vi "Archery_Main.vi"() -> ()   [LabVIEW 2014]
panel:
  in  "Exit":bool
  in  "Cluster":T1
  # "Archery Simulator"
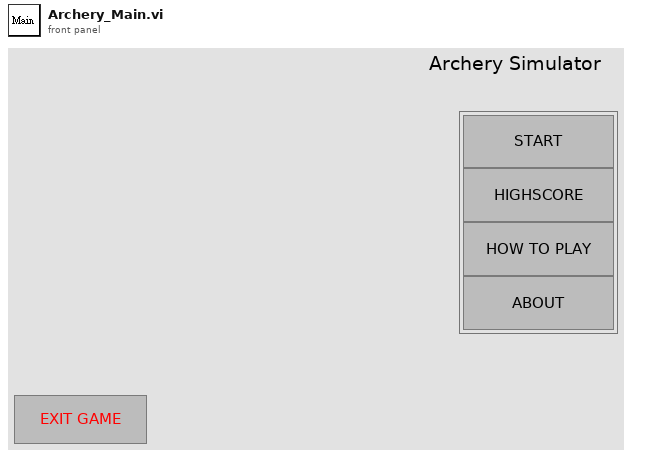
[diagram p1: front panel]
types:
  T1 = cluster{"Start":bool, "Highscore":bool, "Highscore 2":bool, "Highscore 3":bool}
  T2 = enum16{"init", "wait", "game", "highscore", "about", "hint"}
  T3 = enum16{"init", "wait", "game", "highscore", "about"}
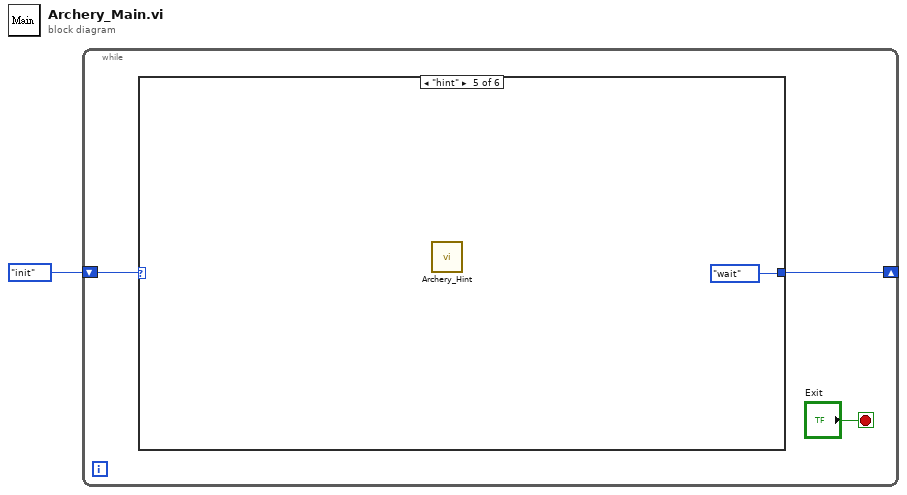
[diagram p0: block diagram]
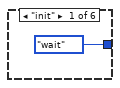
[diagram p2: hidden frame]
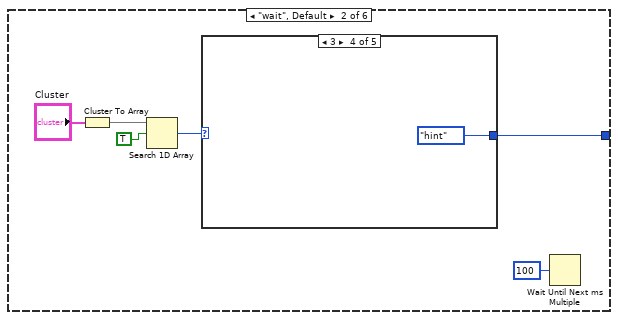
[diagram p3: hidden frame]
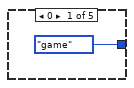
[diagram p4: hidden frame]
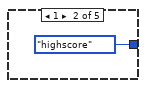
[diagram p5: hidden frame]
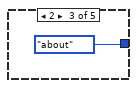
[diagram p6: hidden frame]
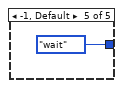
[diagram p7: hidden frame]
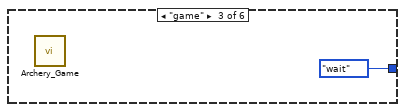
[diagram p8: hidden frame]
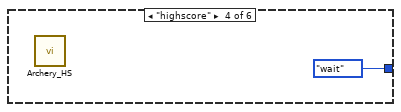
[diagram p9: hidden frame]
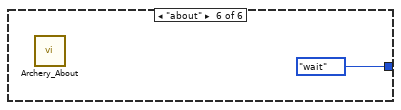
[diagram p10: hidden frame]
diagram:
  n1 = while {
    shift-right: [w3] -> _
    shift-left: T2."init" -> [w4]
    stop <- "Exit" stop-if-true
    n2 = case shown="\"hint\"" w4 {
      tunnel: [enum16{"init", "wait", "game", "highscore"}."wait" w11 enum16{"init", "wait", "game", "highscore"}."wait" enum16{"init", "wait", "game", "highscore"}."wait" T2."wait" T3."wait"] -> w3
      frame "init" {
      }
      frame "wait", Default {
        n3 = Cluster To Array(cluster="Cluster") -> (array=w10:bool[])
        n4 = Search 1D Array(1D array=w10, element=TRUE) -> (index of element=w7:i32)  [unwired: 1 in]
        n5 = case shown="3" w7 {
          tunnel: [enum16{"init", "wait", "game", "highscore"}."game" enum16{"init", "wait", "game", "highscore"}."highscore" T3."about" T2."hint" enum16{"init", "wait", "game", "highscore"}."wait"] -> w11
          frame 0 {
          }
          frame 1 {
          }
          frame 2 {
          }
          frame 3 {
          }
          frame -1, Default {
          }
        }
        n6 = Wait Until Next ms Multiple(millisecond multiple=u32 100) -> ()  [unwired: 1 out]
      }
      frame "game" {
        n7 = call "Archery_Game.vi"() -> ()  [unwired: 12 in]
      }
      frame "highscore" {
        n8 = call "Archery_HS.vi"() -> ()  [unwired: 12 in]
      }
      frame "hint" {
        n9 = call "Archery_Hint.vi"() -> ()  [unwired: 12 in]
      }
      frame "about" {
        n10 = call "Archery_About.vi"() -> ()  [unwired: 4 in]
      }
    }
  }
